vi "Compute Angle.vi"(8 "X Resolution":dbl, 10 "Camera Type":enum16{"206", "1011"}(ring), 11 "X Center (Relative)":dbl) -> (2 "Angle":dbl)   [LabVIEW 2012]
panel:
  in  "Camera view angle":dbl[](array[numeric])=[48.0, 43.5]
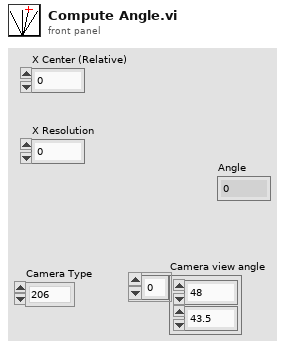
[diagram p1: front panel]
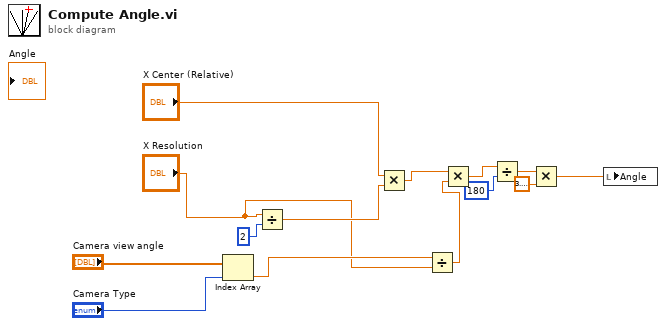
[diagram p0: block diagram]
diagram:
  n1 = Index Array(array="Camera view angle", index="Camera Type") -> (element=w10:dbl)
  n2 = Divide(x="X Resolution", y=2) -> (x/y=w11:dbl)
  n3 = Multiply(x="X Center (Relative)", y=w11) -> (x*y=w8:dbl)
  n4 = Divide(x=w10, y="X Resolution") -> (x/y=w9:dbl)
  n5 = Multiply(x=w8, y=w9) -> (x*y=w5:dbl)
  n6 = Divide(x=w5, y=180) -> (x/y=w3:dbl)
  n7 = Multiply(x=w3, y=3.141592653589793) -> (x*y=w1:dbl)
  n8 = local write "Angle"(w1) -> ()
